vi "IO_Dataq_ReadAIn.vi"(8 "error in (no error)":errorcluster, 10 "Num Chan":i32=2, 11 "VISA Refnum in":refnum<visa-resource-name>="COM3") -> (0 "error out":errorcluster={"status"=FALSE, "code"=1073676294, "source"="VISA Read in IO_Dataq_ReadAIn.vi->_OLS_Main.vi"}, 1 "Outputs":dbl[](array[numeric]), 2 "Waveform Chart":dbl[][](graph), 3 "VISA Refnum out":refnum<visa-resource-name>="COM3", 4 "Bytes at Port":u32=12352)   [LabVIEW 2024]
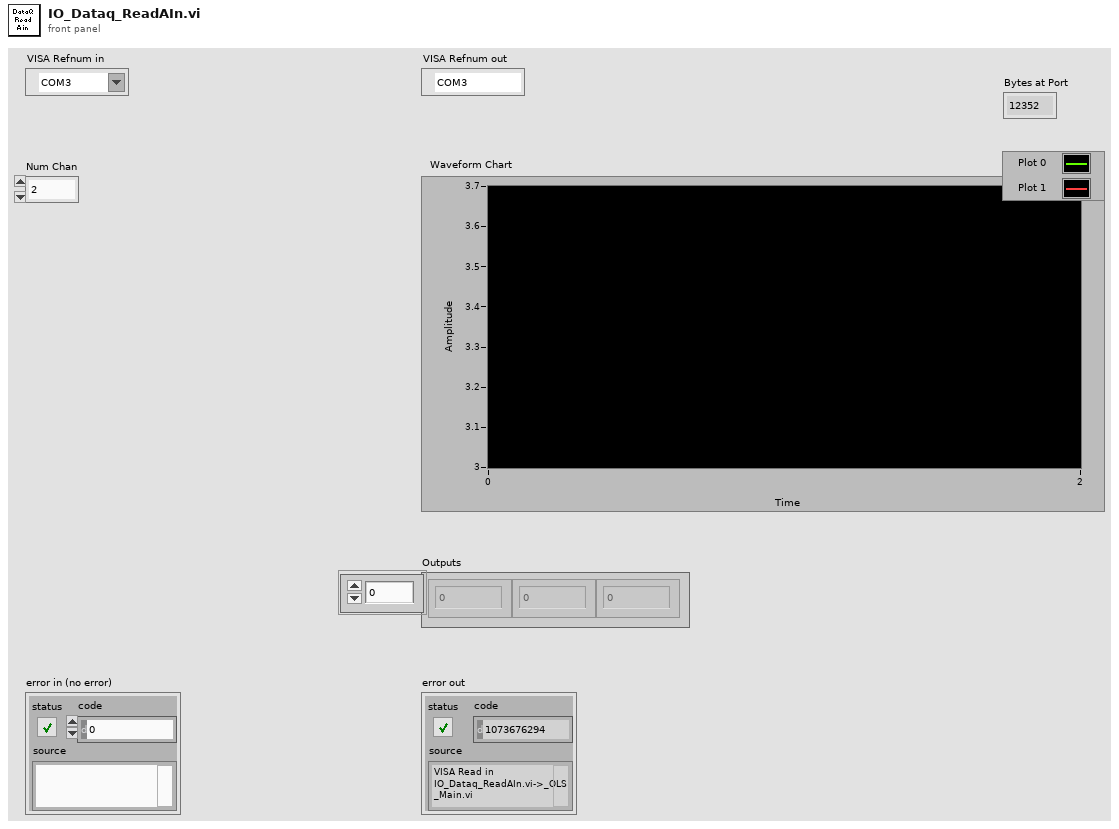
[diagram p1: front panel]
types:
  T1 = enum16{"big-endian, network order", "native, host order", "little-endian"}
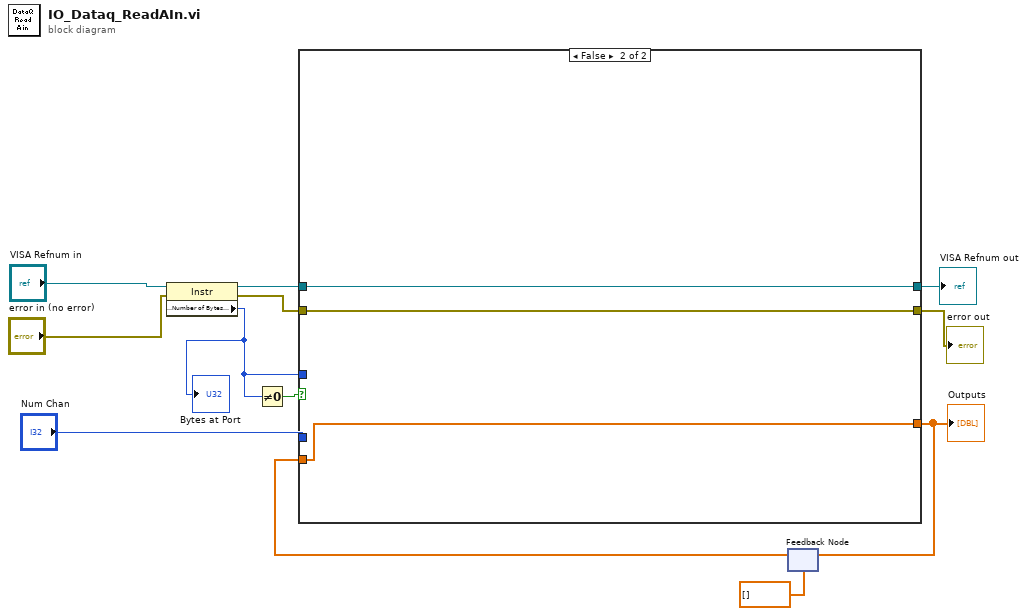
[diagram p0: block diagram]
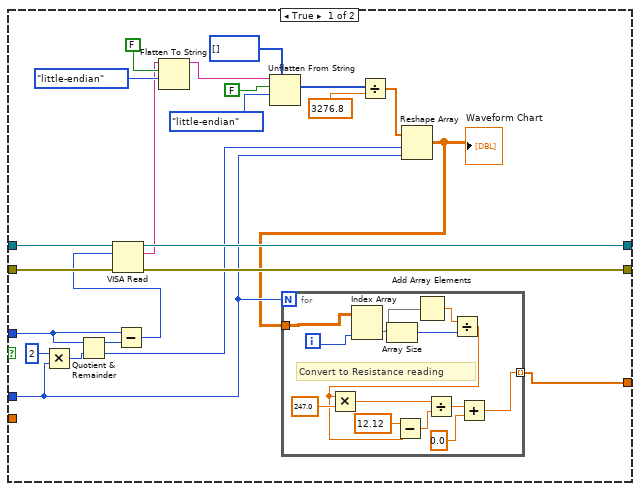
[diagram p2: hidden frame]
diagram:
  n1 = property class="Instr"(reference="VISA Refnum in", error in="error in (no error)") -> (reference out=w7:refnum<visa-resource-name>, error out=w9:errorcluster, "Serial Settings:Number of Bytes at Serial Port"=w10:u32)
  "Bytes at Port" <- w10
  n2 = Not Equal To 0?(x=w10) -> (x != 0?=w11:bool)
  n3 = feedback #1(dbl[] []) -> (w1:dbl[])
  n4 = case shown="False" w11 {
    tunnel: [w34 w50] -> w4
    tunnel: w9 -> [w35 w51]
    tunnel: [w30 w51] -> w5
    tunnel: w7 -> [w17 w50]
    tunnel: w10 -> [w16 _]
    tunnel: "Num Chan" -> [w15 _]
    tunnel: [w13 w49] -> w3
    tunnel: w1 -> [_ w49]
    frame True {
      n5 = Multiply(x=2, y=w15) -> (x*y=w18:i32)
      n6 = Quotient & Remainder(x=w16, y=w18) -> (x-y*floor(x/y)=w32:u32, floor(x/y)=w20:u32)
      n7 = Subtract(x=w16, y=w32) -> (x-y=w31:u32)
      n8 = VISA Read(VISA resource name=w17, byte count=w31, error in (no error)=w35) -> (VISA resource name out=w34:refnum<visa-resource-name>, read buffer=w24:string, error out=w30:errorcluster)  [unwired: 1 out]
      n9 = Flatten To String(anything=w24, prepend array or string size? (T)=FALSE, byte order (0:big-endian, network order)=T1."little-endian") -> (data string=w25:string)  [unwired: 1 in, 2 out]
      n10 = Unflatten From String(type=i16[] [], binary string=w25, data includes array or string size? (T)=FALSE, byte order (0:big-endian, network order)=T1."little-endian") -> (value=w23:i16[])  [unwired: 1 in, 2 out]
      n11 = Divide(x=w23, y=3276.8) -> (x/y=w21:dbl[])
      n12 = Reshape Array(w21, w20, w15) -> (w14:dbl[][])
      "Waveform Chart" <- w14
      n13 = for {
        N: w15 -> [_]
        tunnel: w14 -> [w48]
        tunnel: [w36] -> w13 mode=indexing
        i -> [w44]
        # "Convert to Resistance reading"
        n14 = Index Array(array=w48, index (col)=w44) -> (element=w45:dbl[])  [unwired: 1 in]
        n15 = Array Size(array=w45) -> (size(s)=w46:i32)
        n16 = Add Array Elements(numeric array=w45) -> (sum=w47:dbl)
        n17 = Divide(x=w47, y=w46) -> (x/y=w41:dbl)
        n18 = Multiply(x=w41, y=247.0) -> (x*y=w39:dbl)
        n19 = Subtract(x=12.12, y=w41) -> (x-y=w40:dbl)
        n20 = Divide(x=w39, y=w40) -> (x/y=w38:dbl)
        n21 = Add(x=w38, y=0.0) -> (x+y=w36:dbl)
      }
    }
    frame False {
    }
  }
  "error out" <- w5
  "VISA Refnum out" <- w4
  "Outputs" <- w3
  n22 = feedback-in #1(w3) -> ()
